vi "add set gating(SubVI).vi"(10 "字符串":string) -> (1 "ok or cancel":bool=TRUE, 2 "连接的字符串":string)   [LabVIEW 2019, in "Add Seq.lvlib"]
uses:
  Add Seq.lvlib
panel:
  in  "ok":bool
  in  "cancel":bool
  in  "Amplitude":dbl
  in  "Channel":i32(ring) items=["Channel A", "Channel B"]
  in  "Rate(mV/s)":dbl
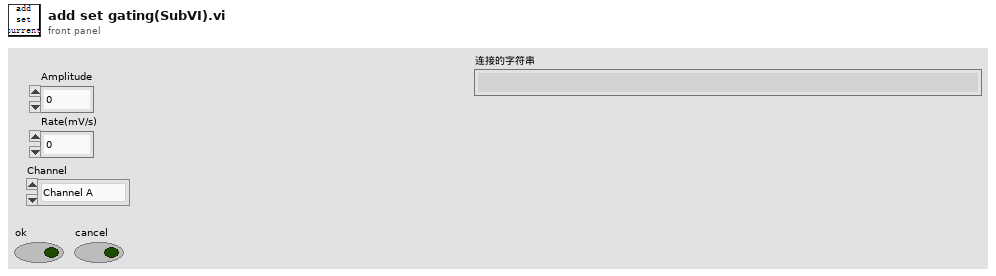
[diagram p1: front panel]
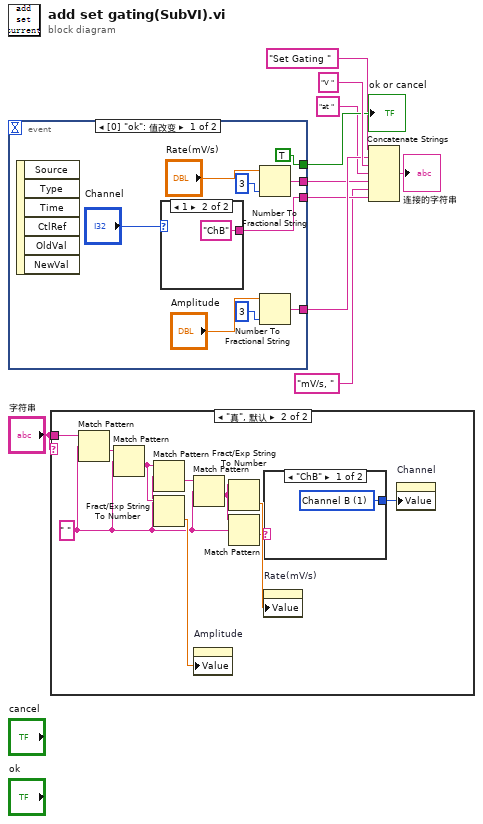
[diagram p0: block diagram]
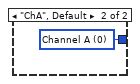
[diagram p3: hidden frame]
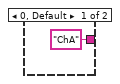
[diagram p4: hidden frame]
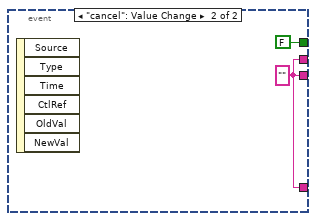
[diagram p5: hidden frame]
diagram:
  n1 = event shown="[0] \"ok\": 值改变" {
    selector: _ -> [_ _]
    dyn-events: _ -> [_ _]
    timeout: _ -> [_ _]
    tunnel: [TRUE FALSE] -> w8
    tunnel: [w14 w22] -> w6
    tunnel: [w13 w22] -> w4
    tunnel: [w12 w22] -> w2
    event "ok": Value Change {
      n2 = event-data() -> ()  [unwired: 1 in, 6 out]
      n3 = case shown="1" "Channel" {
        tunnel: ["ChA" "ChB"] -> w12
        frame 0, Default {
        }
        frame 1 {
        }
      }
      n4 = Number To Fractional String(number="Rate(mV/s)", precision (6)=i16 3 ("精度(6)")) -> (F-format string=w13:string)  [unwired: 2 in]
      n5 = Number To Fractional String(number="Amplitude", precision (6)=i16 3 ("精度(6)")) -> (F-format string=w14:string)  [unwired: 2 in]
    }
    event "cancel": Value Change {
      w22 = ""
      n6 = event-data() -> ()  [unwired: 1 in, 6 out]
    }
  }
  "ok or cancel" <- w8
  n7 = case shown="\"真\", 默认" "字符串" {
    tunnel: "字符串" -> [_ w33]
    frame "" {
    }
    frame "真", Default {
      w27 = " " ("正则表达式")
      n8 = Match Pattern(string=w33, regular expression=w27) -> (after substring=w32:string)  [unwired: 1 in, 3 out]
      n9 = Match Pattern(string=w32, regular expression=w27) -> (after substring=w31:string)  [unwired: 1 in, 3 out]
      n10 = Match Pattern(string=w31, regular expression=w27) -> (after substring=w28:string)  [unwired: 1 in, 3 out]
      n11 = Fract/Exp String To Number(string=w31) -> (number=w30:dbl)  [unwired: 3 in, 1 out]
      n12 = Match Pattern(string=w28, regular expression=w27) -> (after substring=w26:string)  [unwired: 1 in, 3 out]
      n13 = property on="Amplitude" class="DigNum (严格)"("Value"=w30) -> ()  [unwired: 2 in, 2 out]
      n14 = Fract/Exp String To Number(string=w26) -> (number=w29:dbl)  [unwired: 3 in, 1 out]
      n15 = Match Pattern(string=w26, regular expression=w27) -> (after substring=w25:string)  [unwired: 1 in, 3 out]
      n16 = case shown="\"ChB\"" w25 {
        tunnel: [w34 w35] -> w24
        frame "ChB" {
          w34 = 1 items=["Channel A", "Channel B"] ("Channel")
        }
        frame "ChA", Default {
          w35 = 0 items=["Channel A", "Channel B"] ("Channel")
        }
      }
      n17 = property on="Rate(mV/s)" class="DigNum (严格)"("Value"=w29) -> ()  [unwired: 2 in, 2 out]
      n18 = property on="Channel" class="Ring (严格)"("Value"=w24) -> ()  [unwired: 2 in, 2 out]
    }
  }
  n19 = Concatenate Strings("Set Gating " ("字符串"), w6, "V " ("字符串"), "at " ("字符串"), w4, "mV/s, " ("字符串"), w2) -> (→"连接的字符串":string)
